vi "VI-Inherits From KObject.vi"(0 "LVClass Ref":refnum<vi>, 11 "error in (no error)":errorcluster) -> (4 "LVClass Ref out":refnum<vi>, 8 "inherits?":bool, 15 "error out":errorcluster)   [LabVIEW 2020]
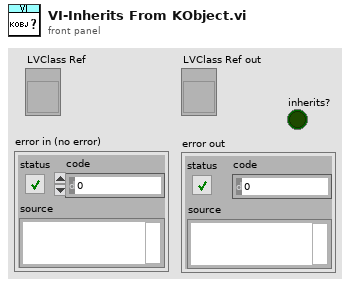
[diagram p1: front panel]
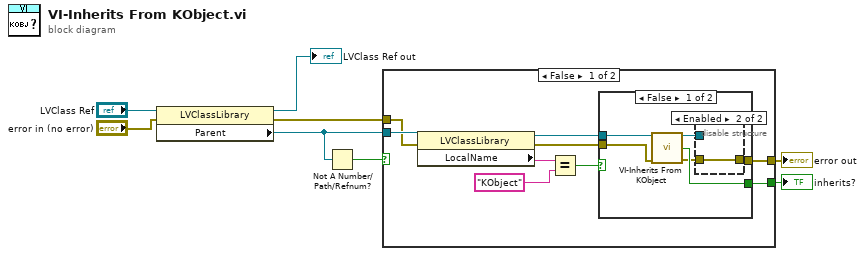
[diagram p0: block diagram]
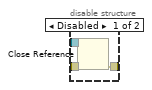
[diagram p2: hidden frame]
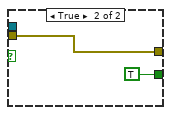
[diagram p3: hidden frame]
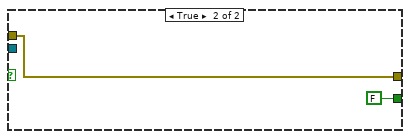
[diagram p4: hidden frame]
diagram:
  n1 = property class="LVClassLibrary"(reference="LVClass Ref", error in="error in (no error)") -> (reference out=→"LVClass Ref out":refnum<vi>, error out=w5:errorcluster, "Parent"=w7:refnum<vi>)
  n2 = Not A Number/Path/Refnum?(number/path/refnum=w7) -> (NaN/Path/Refnum?=w6:bool)
  n3 = case shown="False" w6 {
    tunnel: w7 -> [w15 _]
    tunnel: w5 -> [w14 w30]
    tunnel: [w11 FALSE] -> w4
    tunnel: [w10 w30] -> w3
    frame False {
      n4 = property class="LVClassLibrary"(reference=w15, error in=w14) -> (reference out=w13:refnum<vi>, error out=w9:errorcluster, "LocalName"=w17:string)
      n5 = Equal?(x=w17, y="KObject") -> (x = y?=w12:bool)
      n6 = case shown="False" w12 {
        tunnel: w13 -> [w23 _]
        tunnel: [w21 TRUE] -> w11
        tunnel: [w18 w28] -> w10
        tunnel: w9 -> [w22 w28]
        frame False {
          n7 = call "VI-Inherits From KObject.vi"("LVClass Ref"=w23, "error in (no error)"=w22) -> ("LVClass Ref out"=w20:refnum<vi>, "inherits?"=w21:bool, "error out"=w19:errorcluster)  [unwired: 11 in]
          n8 = disable-structure shown="Enabled" {
            disable-tunnel: w20 -> [w26 _]
            disable-tunnel: w19 -> [w25 w27]
            disable-tunnel: [w24 w27] -> w18
            frame Disabled {
              n9 = Close Reference(reference=w26, error in (no error)=w25) -> (error out=w24:errorcluster)
            }
            frame Enabled {
            }
          }
        }
        frame True {
        }
      }
    }
    frame True {
    }
  }
  "inherits?" <- w4
  "error out" <- w3
